vi "XIPIN_AXI_HWICAP_3_0.vi"   [LabVIEW 2017]
doc: "This core enables an embedded microprocessor, such as the MicroBlaze processor, to read and write the Field Programmable Gate Array (FPGA) configuration memory through the Internal Configuration Access Port (ICAPE2).\n------------------------------------\n<b>Need License</b> : No\n<b>Interface</b> : AXI4"
uses:
  <vilib>/rvi/XilinxIP/XIPIN_XNode/niFpgaXIPIN.xnode
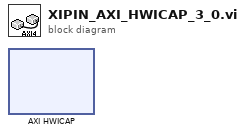
[diagram p0: block diagram]
diagram:
  n1 = xnode ("AXI HWICAP")() -> ()
